vi "afgsafgagSg.vi"() -> ()   [LabVIEW 2019]
uses:
  <vilib>/Math Plots/3D Math Plots/3D Surface/3D Surface XCtrl/3D Surface.xctl
  <vilib>/Utility/miscctls.llb/LVMapReplaceAction.ctl
  9eac16f5-10ab-4925-98c8-b00ca941aca7.vi
  <vilib>/Math Plots/3D Math Plots/3D Surface/3D Surface Datatype/Public/Plot Helper (Vector).vi
  <vilib>/Analysis/NI_AALBase.lvlib
  <vilib>/Math Plots/3D Math Plots/3D Surface/3D Surface Datatype/3D Surface Datatype.lvclass
panel:
  out "output array 2":u32[][](array[numeric])
  out "3D Surface 2":refnum<class "3D Plot Datatype.lvclass">[](xcontrol)
  out "Intensity Graph 2":u32[][](graph)
  out "Numeric":i32
  out "map":map{u32, u32}(c390)
  out "X 2":dbl[](array[numeric])
  out "array with duplicates removed":u32[](array[numeric])
  out "Array":i32[](array[numeric])
  out "Intensity Graph":u32[][](graph)
  out "First Channel":dbl
  out "3D Surface":refnum<class "3D Plot Datatype.lvclass">[](xcontrol)
  out "output array":i32[][](array[numeric])
  out "Histogram Graph":T1(graph)
  in  "Channel":u32[](array[numeric])
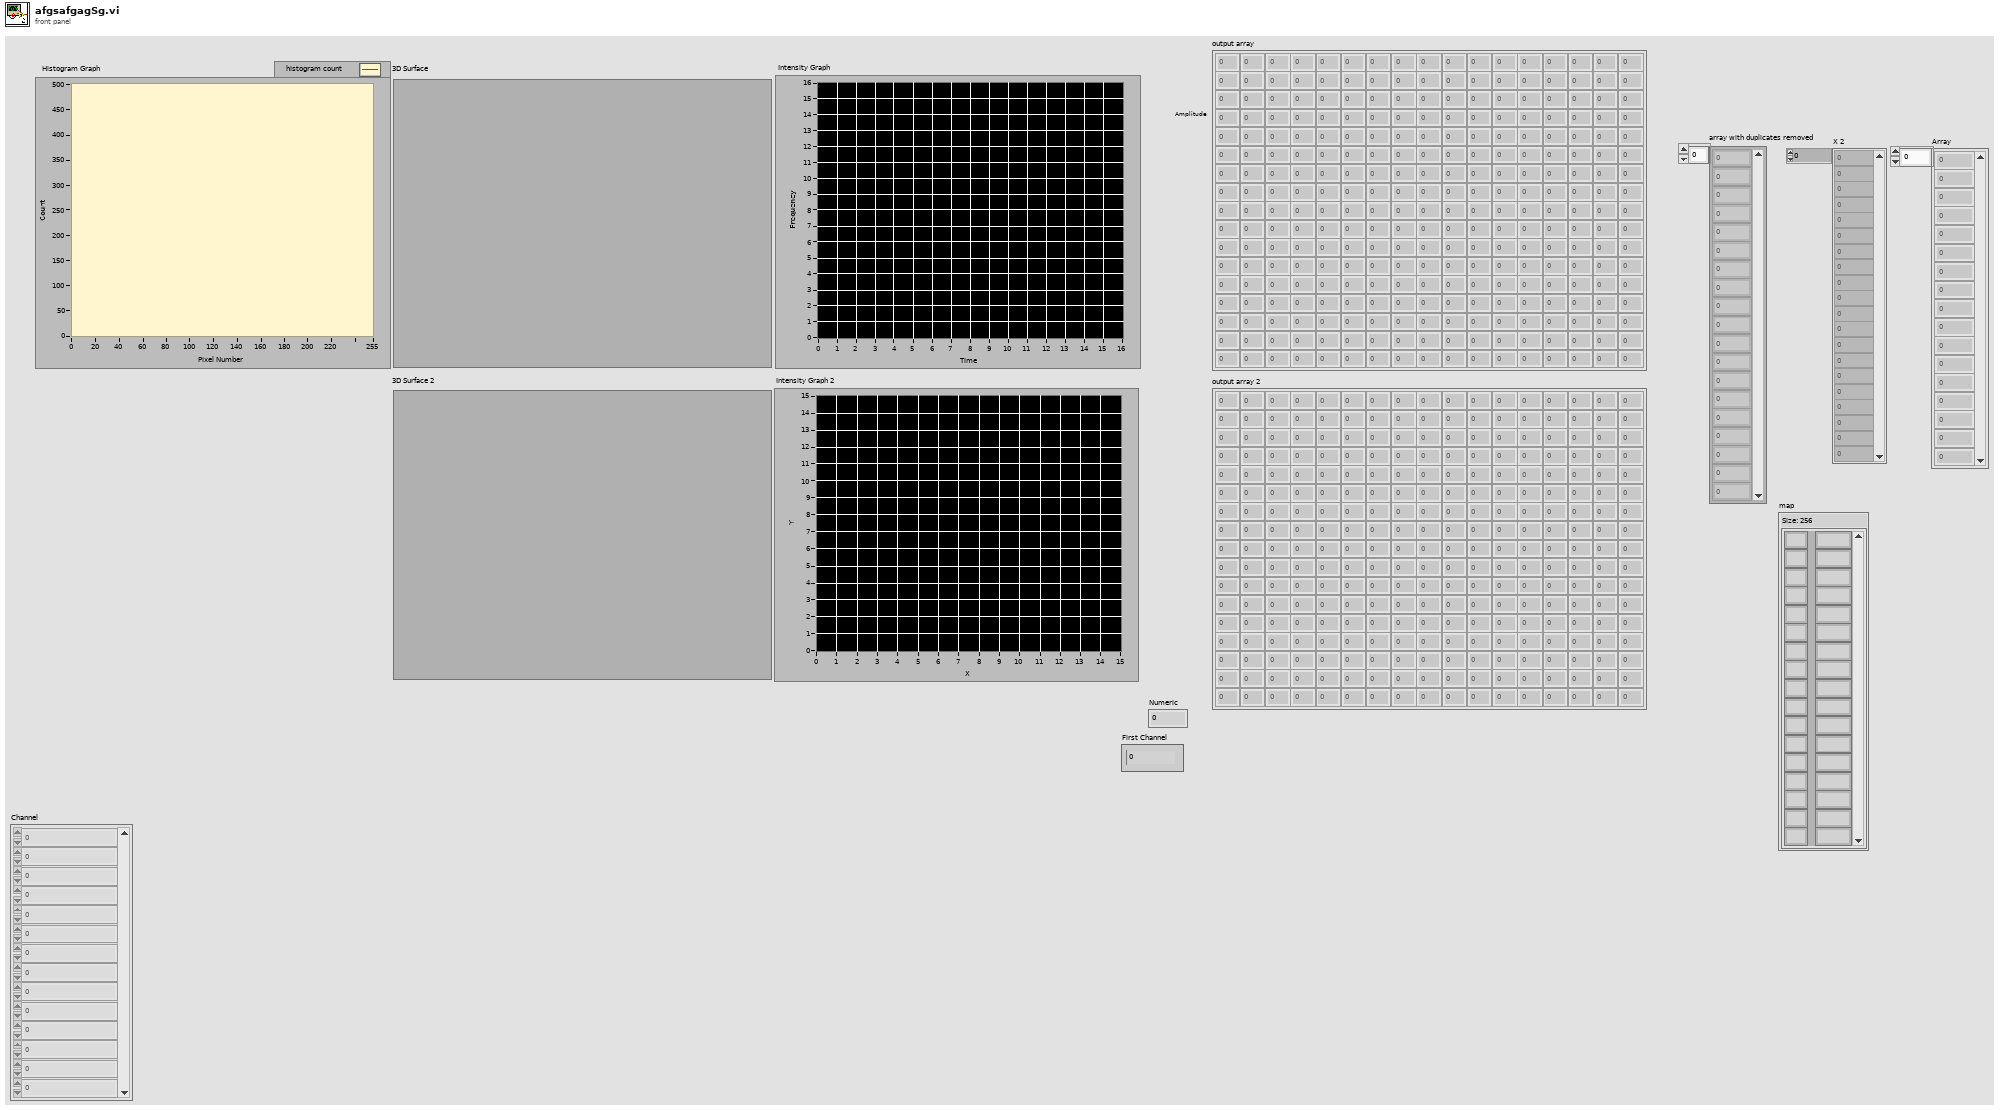
[diagram p1: front panel]
types:
  T1 = cluster{"X Values":dbl[], "Histogram: h(x)":i32[]}
  T2 = typedef "LVMapReplaceAction.ctl" = enum32{"Modify Entry only if found", "Add or Modify Entry", "Delete Entry"}
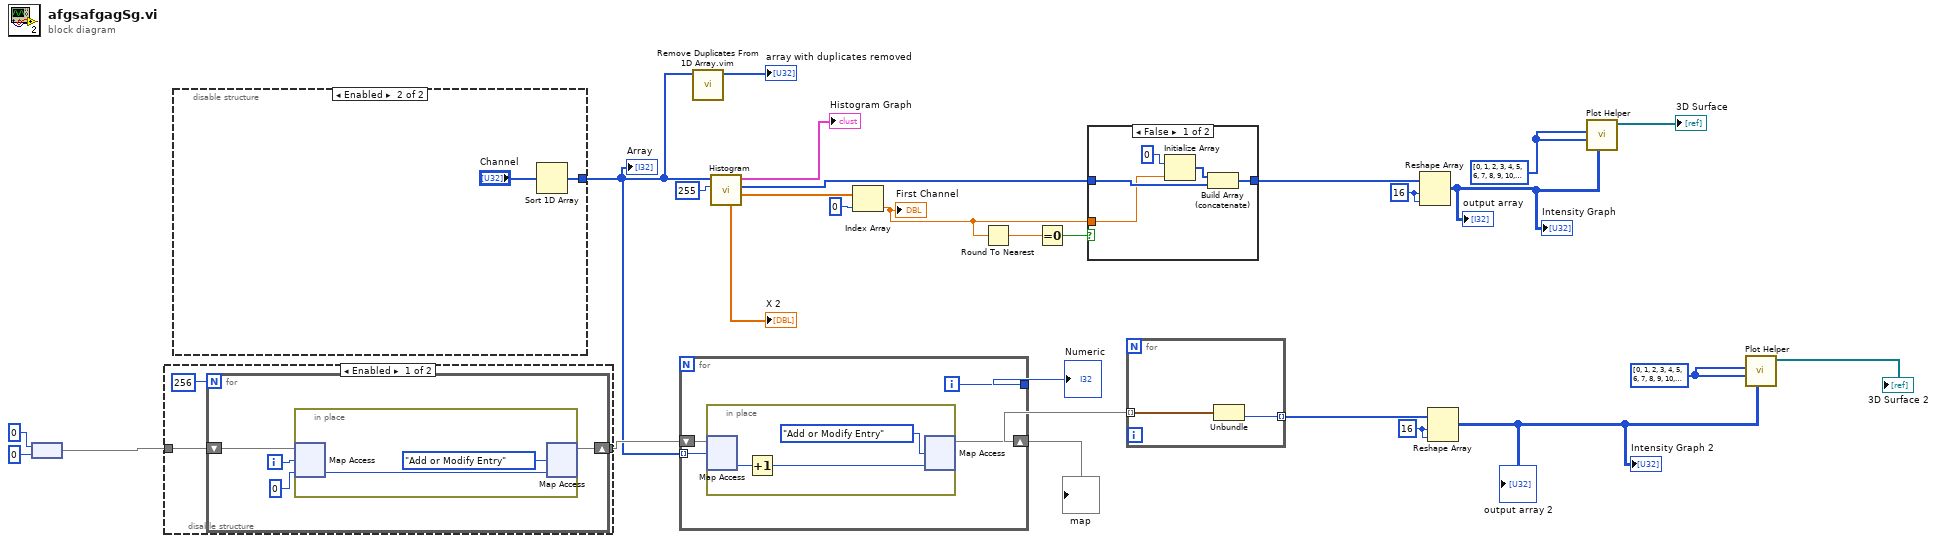
[diagram p0: block diagram]
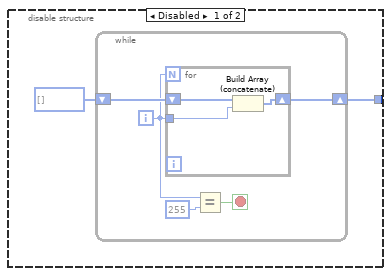
[diagram p4: hidden frame]
diagram:
  w3 = u8[] [0, 1, 2, 3, 4, 5, 6, 7, 8, 9, 10, 11, 12, 13, 14, 15, 0, 1, 2, 3, 4, 5, 6, 7, 8, 9, 10, 11, 12, 13, 14, 15, 0, 1, 2, 3, 4, 5, 6, 7, 8, 9, 10, 11, 12, 13, 14, 15, 0, 1, 2, 3, 4, 5, 6, 7, 8, 9, 10, 11, 12, 13, 14, 15, 0, 1, 2, 3, 4, 5, 6, 7, 8, 9, 10, 11, 12, 13, 14, 15, 0, 1, 2, 3, 4, 5, 6, 7, 8, 9, 10, 11, 12, 13, 14, 15, 0, 1, 2, 3, 4, 5, 6, 7, 8, 9, 10, 11, 12, 13, 14, 15, 0, 1, 2, 3, 4, 5, 6, 7, 8, 9, 10, 11, 12, 13, 14, 15, 0, 1, 2, 3, 4, 5, 6, 7, 8, 9, 10, 11, 12, 13, 14, 15, 0, 1, 2, 3, 4, 5, 6, 7, 8, 9, 10, 11, 12, 13, 14, 15, 0, 1, 2, 3, 4, 5, 6, 7, 8, 9, 10, 11, 12, 13, 14, 15, 0, 1, 2, 3, 4, 5, 6, 7, 8, 9, 10, 11, 12, 13, 14, 15, 0, 1, 2, 3, 4, 5, 6, 7, 8, 9, 10, 11, 12, 13, 14, 15, 0, 1, 2, 3, 4, 5, 6, 7, 8, 9, 10, 11, 12, 13, 14, 15, 0, 1, 2, 3, 4, 5, 6, 7, 8, 9, 10, 11, 12, 13, 14, 15, 0, 1, 2, 3, 4, 5, 6, 7, 8, 9, 10, 11, 12, 13, 14] ("Array")
  w4 = 16
  w20 = u8[] [0, 1, 2, 3, 4, 5, 6, 7, 8, 9, 10, 11, 12, 13, 14, 15, 0, 1, 2, 3, 4, 5, 6, 7, 8, 9, 10, 11, 12, 13, 14, 15, 0, 1, 2, 3, 4, 5, 6, 7, 8, 9, 10, 11, 12, 13, 14, 15, 0, 1, 2, 3, 4, 5, 6, 7, 8, 9, 10, 11, 12, 13, 14, 15, 0, 1, 2, 3, 4, 5, 6, 7, 8, 9, 10, 11, 12, 13, 14, 15, 0, 1, 2, 3, 4, 5, 6, 7, 8, 9, 10, 11, 12, 13, 14, 15, 0, 1, 2, 3, 4, 5, 6, 7, 8, 9, 10, 11, 12, 13, 14, 15, 0, 1, 2, 3, 4, 5, 6, 7, 8, 9, 10, 11, 12, 13, 14, 15, 0, 1, 2, 3, 4, 5, 6, 7, 8, 9, 10, 11, 12, 13, 14, 15, 0, 1, 2, 3, 4, 5, 6, 7, 8, 9, 10, 11, 12, 13, 14, 15, 0, 1, 2, 3, 4, 5, 6, 7, 8, 9, 10, 11, 12, 13, 14, 15, 0, 1, 2, 3, 4, 5, 6, 7, 8, 9, 10, 11, 12, 13, 14, 15, 0, 1, 2, 3, 4, 5, 6, 7, 8, 9, 10, 11, 12, 13, 14, 15, 0, 1, 2, 3, 4, 5, 6, 7, 8, 9, 10, 11, 12, 13, 14, 15, 0, 1, 2, 3, 4, 5, 6, 7, 8, 9, 10, 11, 12, 13, 14, 15, 0, 1, 2, 3, 4, 5, 6, 7, 8, 9, 10, 11, 12, 13, 14] ("Array")
  w25 = 16
  n1 = node(u32 0, u32 0 ("value")) -> (w10:map{u32, u32})
  n2 = disable-structure shown="Enabled" {
    disable-tunnel: w10 -> [w30 w37]
    disable-tunnel: [w29 w37] -> w9
    frame Enabled {
      n3 = for {
        N: 256 -> [_]
        shift-right: [w31] -> w29
        shift-left: w30 -> [w34]
        i -> [w33]
        n4 = in-place {
          n5 = in-place-map #1(w34, w33, 0) -> (w35:u32)  [unwired: 1 out]
          n6 = in-place-map #1(w35, LVMapReplaceAction."Add or Modify Entry" ("action")) -> (w31:map{u32, u32})  [unwired: 2 out]
        }
      }
    }
    frame Disabled {
    }
  }
  n7 = disable-structure shown="Enabled" {
    disable-tunnel: [w38 w48] -> w8
    frame Disabled {
      n8 = while {
        shift-right: [w41] -> w38
        shift-left: i32[] [] -> [w44]
        i -> [w40]
        stop <- w42 stop-if-true
        n9 = for {
          N: w40 -> [_]
          tunnel: w40 -> [w46]
          shift-right: [w45] -> w41
          shift-left: w44 -> [w47]
          n10 = Build Array (concatenate)(w47, w46) -> (w45:i32[])
        }
        n11 = Equal?(x=w40, y=255) -> (x = y?=w42:bool)
      }
    }
    frame Enabled {
      n12 = Sort 1D Array(array="Channel") -> (sorted array=w48:u32[])
    }
  }
  "Array" <- w8
  n13 = for {
    shift-right: [w52] -> w6
    shift-left: w9 -> [w53]
    tunnel: w8 -> [w51] mode=indexing
    tunnel: [w50] -> w7
    i -> [w50]
    n14 = in-place {
      n15 = in-place-map #2(w53, w51) -> (w55:u32)  [unwired: 1 in, 1 out]
      n16 = Increment(x=w55) -> (x+1=w54:u32)
      n17 = in-place-map #2(w54, LVMapReplaceAction."Add or Modify Entry" ("action")) -> (w52:map{u32, u32})  [unwired: 2 out]
    }
  }
  "map" <- w6
  "Numeric" <- w7
  n18 = call "Remove Duplicates From 1D Array.vim"("array"=w8) -> ("array with duplicates removed"=→"array with duplicates removed":u32[])  [unwired: 10 in]
  n19 = call <vilib>:"Histogram.vi"("intervals"=255, "X"=w8) -> ("X Values"=w23:dbl[], "Histogram: h(x)"=w19:i32[], "Histogram Graph"=→"Histogram Graph":T1, "X 2"=→"X 2":dbl[])  [unwired: 5 in, 1 out]
  n20 = Index Array(array=w23, index=u32 0 ("element")) -> (element=w17:dbl)
  "First Channel" <- w17
  n21 = Round To Nearest(number=w17) -> (nearest integer value=w16:dbl)
  n22 = Equal To 0?(x=w16) -> (x = 0?=w15:bool)
  n23 = case shown="False" w15 {
    tunnel: [w60 w62] -> w13
    tunnel: w19 -> [w59 w62]
    tunnel: w17 -> [w58 _]
    frame False {
      n24 = Initialize Array(u32 0 ("element"), w58) -> (w61:u32[])
      n25 = Build Array (concatenate)(w61, w59) -> (w60:u32[])
    }
    frame True {
    }
  }
  n26 = for {
    tunnel: w6 -> [w64] mode=indexing
    tunnel: [w63] -> w5 mode=indexing
    n27 = Unbundle(w64) -> ("value"=w63:u32)  [unwired: 1 out]
  }
  n28 = Reshape Array(w13, w25, w25) -> (w21:u32[][])
  "output array" <- w21
  "Intensity Graph" <- w21
  n29 = Reshape Array(w5, w4, w4) -> (w1:u32[][])
  "Intensity Graph 2" <- w1
  "output array 2" <- w1
  n30 = call-poly <vilib>:"Plot Helper.vi"("z matrix"=w21, "y vector"=w20, "x vector"=w20) -> ("3D Plot lvclass Array out"=→"3D Surface":refnum<class "3D Plot Datatype.lvclass">[])  [unwired: 3 in, 5 out]
  n31 = call-poly <vilib>:"Plot Helper.vi"("z matrix"=w1, "y vector"=w3, "x vector"=w3) -> ("3D Plot lvclass Array out"=→"3D Surface 2":refnum<class "3D Plot Datatype.lvclass">[])  [unwired: 3 in, 5 out]
